vi "write_acq_time.vi"(8 "error in (no error)":errorcluster, 10 "acq_time_s":i32, 11 "tt20 in":refnum<class "tt20.lvclass">) -> (0 "error out":errorcluster, 3 "tt20 out":refnum<class "tt20.lvclass">)   [LabVIEW 2015, in "tt20.lvclass"]
uses:
  tt20.lvclass
  tt20.lvclass/tt20.ctl
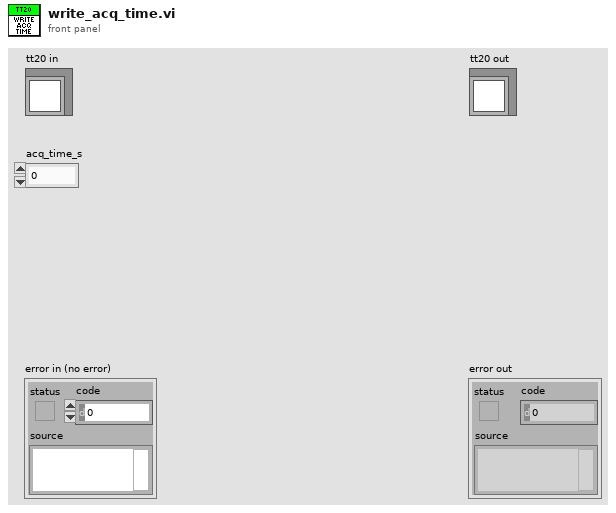
[diagram p1: front panel]
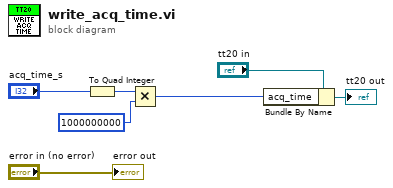
[diagram p0: block diagram]
diagram:
  n1 = To Quad Integer(1:"acq_time_s") -> (0:w1:i64)
  n2 = Multiply(x=w1, y=i64 1000000000) -> (x*y=w3:i64)
  n3 = Bundle By Name(cluster="tt20 in", "acq_time"=w3) -> (→"tt20 out":refnum<class "tt20.lvclass">)
  "error out" <- "error in (no error)"
